vi "projeödevi.vi"() -> ()   [LabVIEW 2017]
uses:
  <vilib>/Utility/NIReport.llb/Append Text Table to Report (wrap).vi
  <vilib>/Utility/NIReport.llb/NI_report.lvclass
  <vilib>/Utility/NIReport.llb/Excel/NI_Excel.lvclass
panel:
  in  "Path":path
  in  "Hasta durumu":string
  in  "KAYIT AL":bool
  in  "stop":bool
  in  "TARİH":timestamp
  in  "NUMARA":dbl
  in  "doktor adı soyadı":string
  in  "Hasta Adı soyadı":string
  out "TABLO":string[][](table)
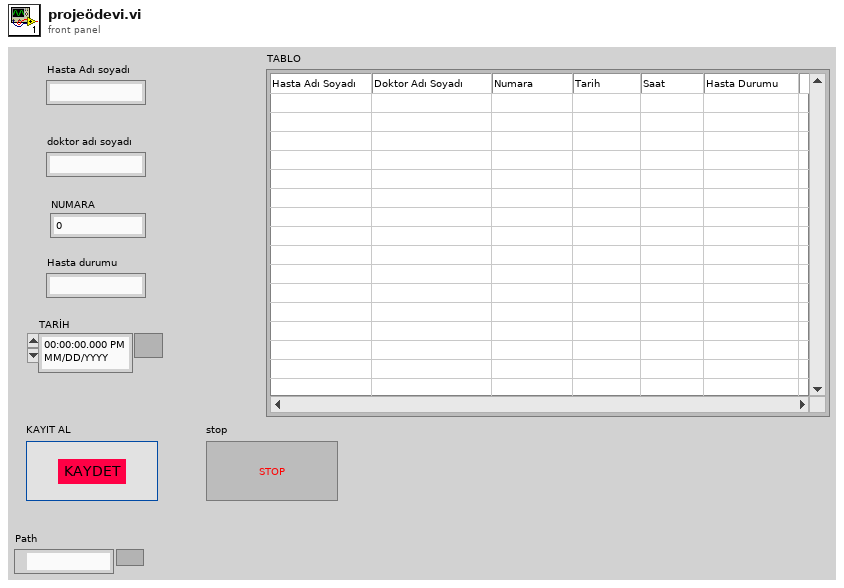
[diagram p1: front panel]
types:
  T1 = enum16{"Standard Report", "HTML", "Word", "Excel"}
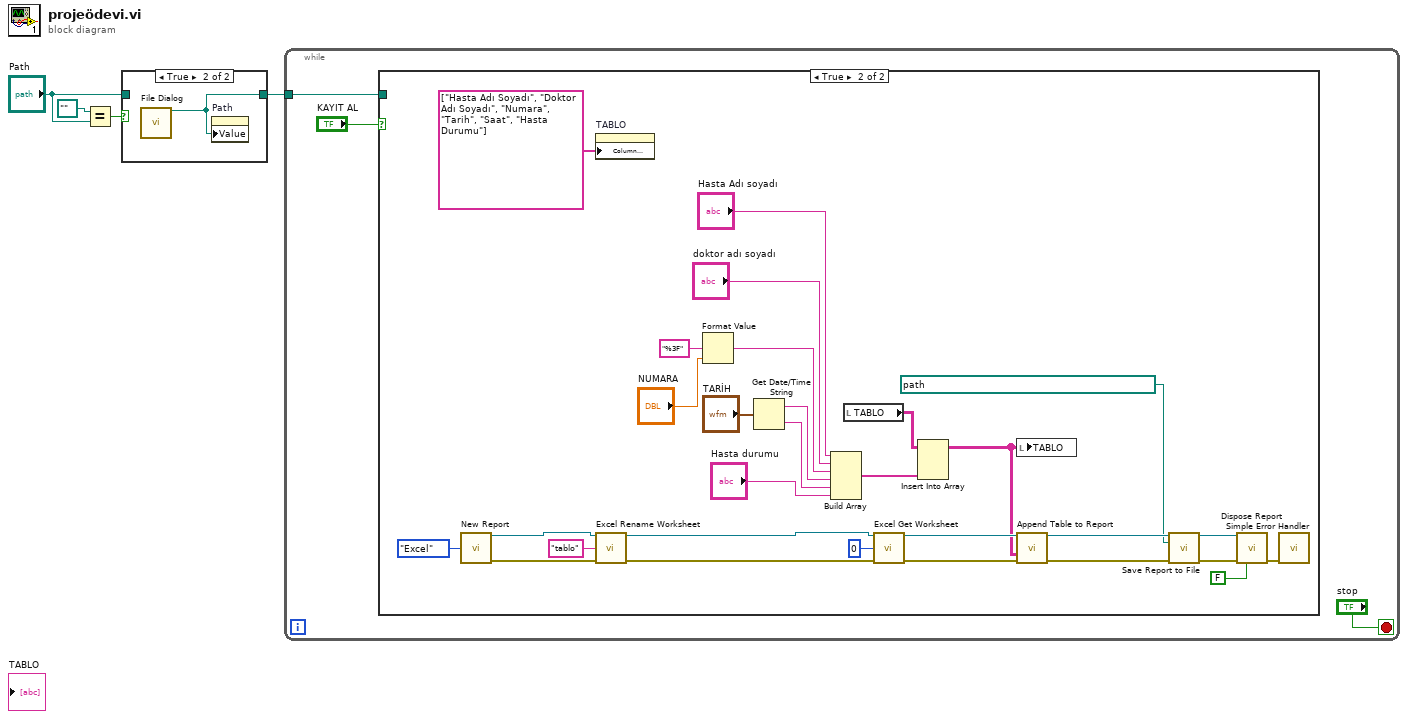
[diagram p0: block diagram]
diagram:
  n1 = Equal?(x=path "", y="Path") -> (x = y?=w3:bool)
  n2 = case shown="True" w3 {
    tunnel: "Path" -> [w5 _]
    tunnel: [w5 w6] -> w2
    frame False {
    }
    frame True {
      n3 = call "File Dialog"() -> ("selected path"=w6:path)  [unwired: 12 in, 3 out]
      n4 = property on="Path" class="Path"("Value"=w6) -> ()  [unwired: 2 in, 2 out]
    }
  }
  n5 = while {
    tunnel: w2 -> [w7]
    stop <- "stop" stop-if-true
    n6 = case shown="True" "KAYIT AL" {
      tunnel: w7 -> [_ _]
      frame False {
      }
      frame True {
        n7 = call <vilib>:"New Report.vi"("report type"=T1."Excel") -> ("report out"=w26:refnum<class "NI_report.lvclass">, "error out"=w25:errorcluster)  [unwired: 13 in]
        n8 = property on="TABLO" class="Tbl (strict)"("Column Headers[]"=string[] ["Hasta Adı Soyadı", "Doktor Adı Soyadı", "Numara", "Tarih", "Saat", "Hasta Durumu"] ("Column Header Strings[]")) -> ()  [unwired: 2 in, 2 out]
        n9 = call <vilib>:"Excel Rename Worksheet.vi"("report in"=w26, "worksheet name (\"\")"="tablo" ("worksheet name (\"\")"), "error in (no error)"=w25) -> ("report out"=w24:refnum<class "NI_report.lvclass">, "error out"=w23:errorcluster)  [unwired: 11 in]
        n10 = Format Value(format string="%3F", value (0)="NUMARA") -> (output string=w35:string)  [unwired: 1 in]
        n11 = Get Date/Time String(seconds (now)="TARİH") -> (date string=w33:string, time string=w32:string)  [unwired: 2 in]
        n12 = Build Array "Build Array"("Hasta Adı soyadı", "doktor adı soyadı", w35, w33, w32, "Hasta durumu") -> (w27:string[])
        n13 = local read "TABLO"() -> (w31:string[][])
        n14 = call <vilib>:"Excel Get Worksheet.vi"("report in"=w24, "worksheet index (0)"=0, "error in (no error)"=w23) -> ("report out"=w22:refnum<class "NI_report.lvclass">, "error out"=w21:errorcluster)  [unwired: 11 in]
        n15 = Insert Into Array "Insert Into Array"(array=w31, new element=w27) -> (w17:string[][])  [unwired: 2 in]
        n16 = local write "TABLO"(w17) -> ()
        n17 = call-poly <vilib>:"Append Table to Report.vi"("report in"=w22, "text data"=w17, "error in (no error)"=w21) -> ("report out"=w16:refnum<class "NI_report.lvclass">, "error out"=w15:errorcluster)  [unwired: 9 in, 2 out]
        n18 = call-dynamic "Save Report to File.vi"("report in"=w16, "report file path"=path "C:/Users/hp/Desktop/Yeni klasör (2)/kayıt.xlsx", "error in (no error)"=w15) -> ("report out"=w14:refnum<class "NI_report.lvclass">, "error out"=w13:errorcluster)  [unwired: 11 in]
        n19 = call-dynamic "Dispose Report.vi"("report in"=w14, "error in (no error)"=w13, "close report? (T)"=FALSE) -> ("error out"=w11:errorcluster)  [unwired: 12 in]
        n20 = call <vilib>:"Simple Error Handler.vi"("error in (no error)"=w11) -> ()  [unwired: 4 in, 5 out]
      }
    }
  }
